vi "Check Lowbar Cross.vi"() -> (3 "Cross":bool)   [LabVIEW 2015]
uses:
  Robot Values.vi
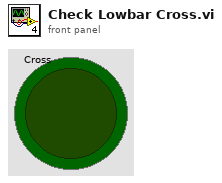
[diagram p1: front panel]
types:
  T1 = typedef "Robot Values.ctl" = cluster{"Drive Motors":cluster{"Left Motor Value":dbl, "Right Motor Value":dbl, "Left Motor Encoder":dbl, "Right Motor Encoder":dbl, "High/Low Gear":bool}, "Sensors":cluster{"Gyro Angle":dbl, "Photoeye":bool, "Ultrasonic Range":dbl, "Shooter Speed Encoder":dbl, "Accelerometer Value":dbl, "Flashlight":bool, "Target Distance":dbl, "Target X Value":dbl, "Reset Gyro?":bool}, "Arms":cluster{"Desired Arm Position":dbl, "Left Arm Encoder":dbl, "Right Arm Encoder":dbl, "Left Arm Lower Limit":bool, "Right Arm Lower Limit":bool, "Initialize Arm Position?":bool}, "Acquisition and Scoring":cluster{"Acquiring?":bool, "Current Speed":dbl, "Setpoint Speed":dbl, "Prep Wheels":bool, "Shoot":bool, "Low Eject":bool, "Reverse Shooter Wheel":bool}, "Hanging":cluster{"Pivot Arms":dbl, "PTO":bool, "Left Pivot Encoder":dbl, "Right Pivot Encoder":dbl, "Hanging Pin":bool}}
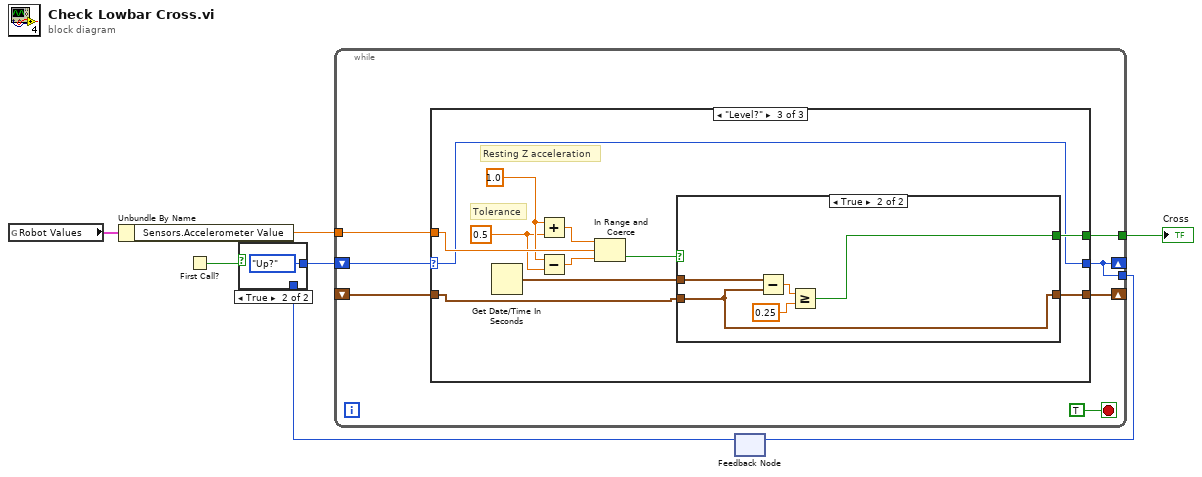
[diagram p0: block diagram]
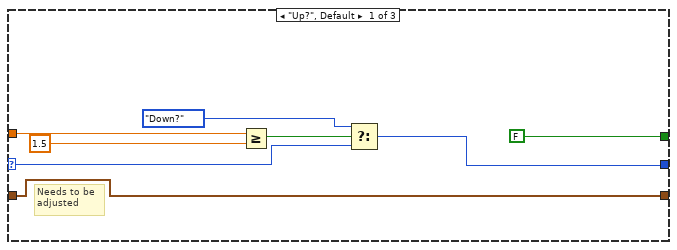
[diagram p3: hidden frame]
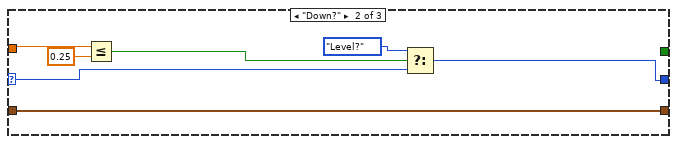
[diagram p4: hidden frame]
diagram:
  n1 = global read "Robot Values.vi" "Robot Values"() -> (w7:T1)
  n2 = Unbundle By Name(w7) -> ("Sensors.Accelerometer Value"=w5:dbl)
  n3 = First Call?() -> (First Call?: T/F=w3:bool)
  n4 = feedback #1() -> (w1:enum16{"Level?", "Up?", "Down?"})  [unwired: 1 in]
  n5 = case shown="True" w3 {
    tunnel: [w8 enum16{"Level?", "Up?", "Down?"}."Up?"] -> w6
    tunnel: w1 -> [w8 _]
    frame False {
    }
    frame True {
    }
  }
  n6 = while {
    shift-right: [w10] -> _
    shift-left: w6 -> [w15]
    tunnel: w5 -> [w14]
    tunnel: [w13] -> w4
    shift-right: [w12] -> _
    shift-left: _ -> [w11]
    tunnel: [w10] -> w2
    stop <- TRUE stop-if-true
    n7 = case shown="\"Level?\"" w15 {
      selector: w15 -> [w22 w25 w36]
      tunnel: [w21 w27 w36] -> w10
      tunnel: w14 -> [w20 w30 w37]
      tunnel: [FALSE _ w39] -> w13
      tunnel: [w17 w26 w41] -> w12
      tunnel: w11 -> [w17 w26 w40]
      frame "Up?", Default {
        # "Needs to be \nadjusted"
        n8 = Greater Or Equal?(x=w20, y=1.5) -> (x >= y?=w23:bool)
        n9 = Select(t=enum16{"Level?", "Up?", "Down?"}."Down?", s=w23, f=w22) -> (s? t:f=w21:enum16{"Level?", "Up?", "Down?"})
      }
      frame "Down?" {
        n10 = Less Or Equal?(x=w30, y=0.25) -> (x <= y?=w29:bool)
        n11 = Select(t=enum16{"Level?", "Up?", "Down?"}."Level?", s=w29, f=w25) -> (s? t:f=w27:enum16{"Level?", "Up?", "Down?"})
      }
      frame "Level?" {
        w32 = 0.5
        w33 = 1.0
        # "Tolerance"
        # "Resting Z acceleration"
        n12 = Get Date/Time In Seconds() -> (seconds since 1Jan1904=w42:timestamp)
        n13 = Add(x=w33, y=w32) -> (x+y=w35:dbl)
        n14 = Subtract(x=w33, y=w32) -> (x-y=w34:dbl)
        n15 = In Range and Coerce(upper limit=w35, x=w37, lower limit=w34) -> (In Range?=w38:bool)  [unwired: 1 out]
        n16 = case shown="True" w38 {
          tunnel: w42 -> [w43 w48]
          tunnel: [w43 w44] -> w41
          tunnel: w40 -> [_ w44]
          tunnel: [_ w45] -> w39
          frame False {
          }
          frame True {
            n17 = Subtract(x=w48, y=w44) -> (x-y=w47:dbl)
            n18 = Greater Or Equal?(x=w47, y=0.25) -> (x >= y?=w45:bool)
          }
        }
      }
    }
  }
  "Cross" <- w4
  n19 = feedback-in #1(w2) -> ()
